vi "Read AJ error Info Table.vi"(8 "error in (no error)":errorcluster, 10 "s":bool, 11 "Linename":string) -> (0 "error IO":errorcluster, 1 "size(s)":i32, 2 "Error BG":u32(colorbox), 3 "Array":string[](array[string]))   [LabVIEW 2014]
uses:
  <vilib>/addons/database/NI_Database_API.lvlib
  <vilib>/addons/database/Connection.llb/DB Tools Open Connec (String).vi
  <vilib>/addons/database/_DB Variant To Data/Database Variant To Data.xnode
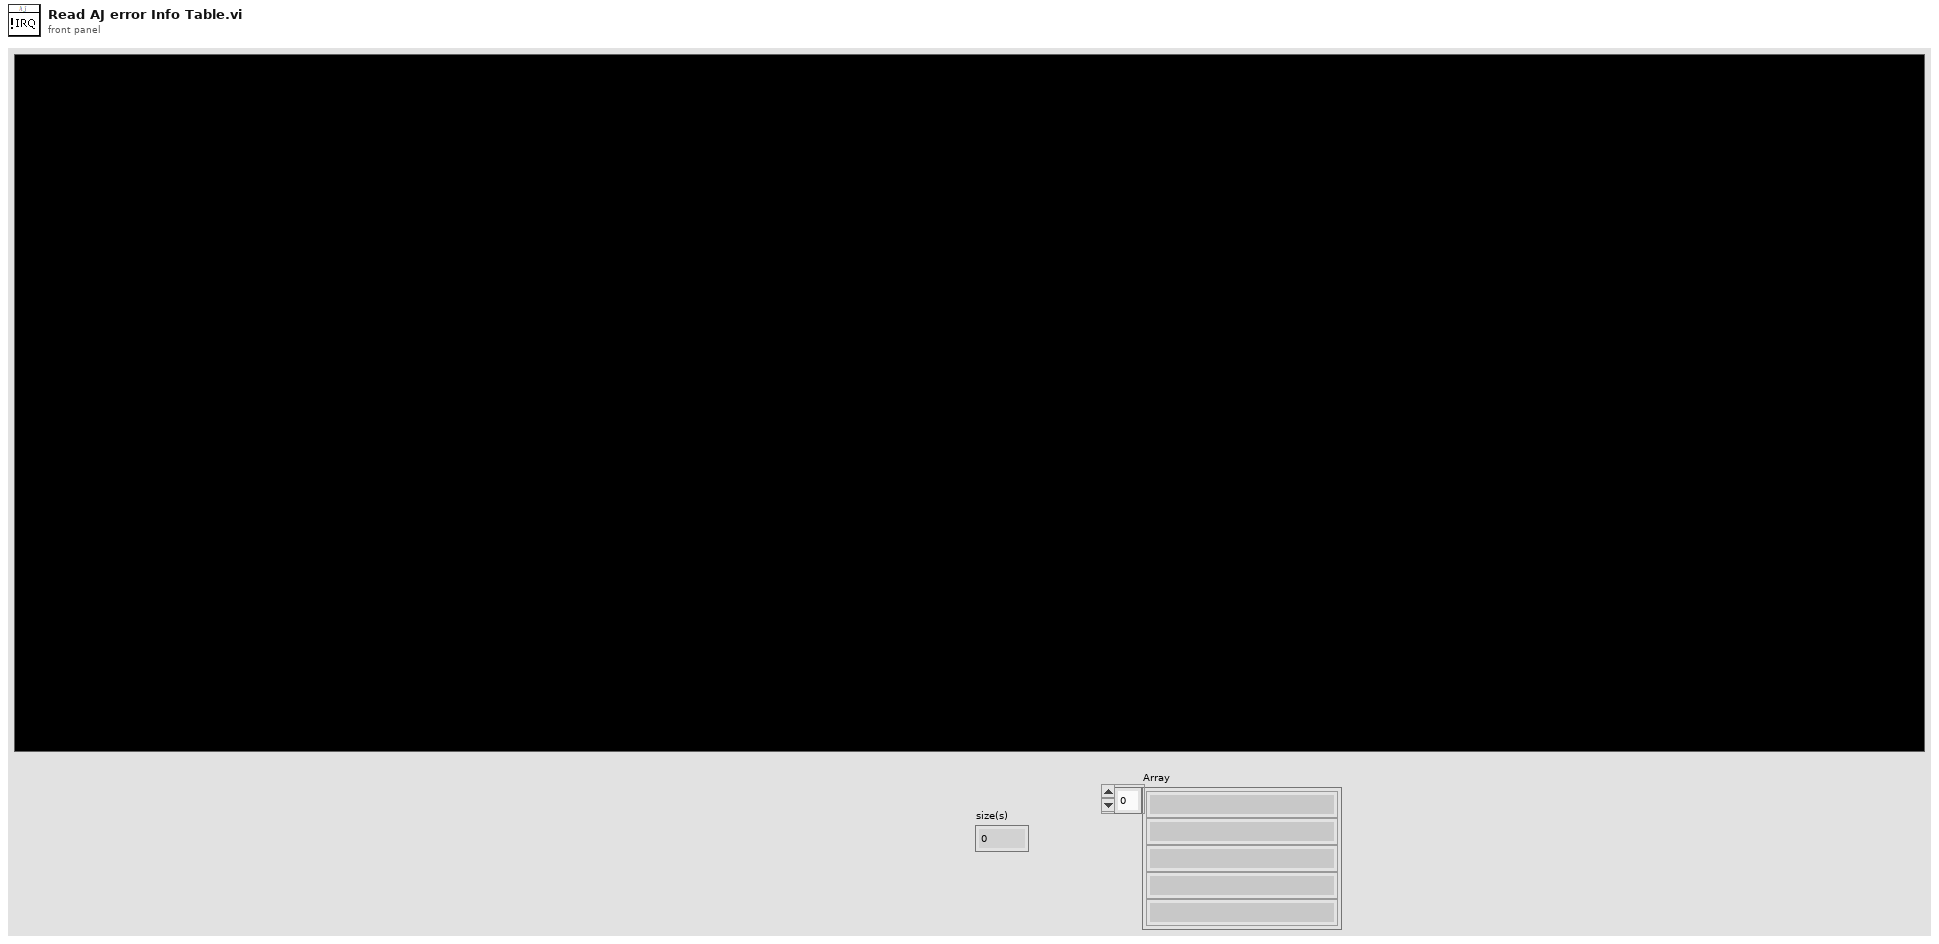
[diagram p1: front panel]
types:
  T1 = cluster{"linename":string, "Stationname":string, "Display Info":string, "startTime":timestamp}[]
  T2 = typedef "NI_Database_API.lvlib/Conn ObjectReference.ctl" = refnum<k1>
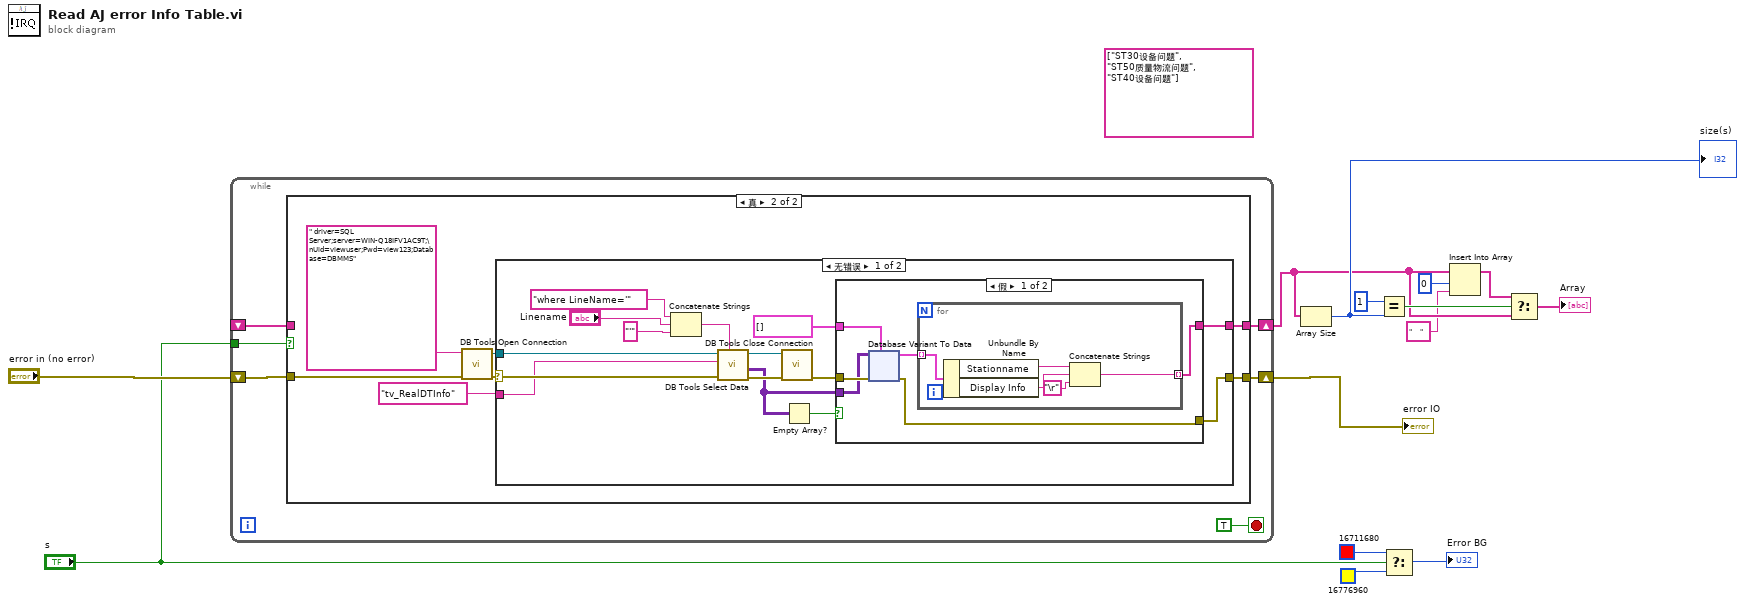
[diagram p0: block diagram]
diagram:
  (unwired) string[] ["ST30设备问题", "ST50质量物流问题", "ST40设备问题"]
  n1 = while {
    tunnel: "s" -> [w15]
    shift-right: [w19] -> w10
    shift-left: "error in (no error)" -> [w20]
    shift-right: [w18] -> w2
    shift-left: _ -> [w16]
    stop <- TRUE stop-if-true
    n2 = case shown="真" w15 {
      tunnel: w20 -> [w21 w28]
      tunnel: [w21 w27] -> w19
      tunnel: [w22 w23] -> w18
      tunnel: w16 -> [w22 _]
      frame False {
      }
      frame True {
        n3 = call-poly <vilib>:"DB Tools Open Connection.vi"("error in (no error)"=w28, "connection information"=" driver=SQL Server;server=WIN-Q18IFV1AC9T;\nUid=viewuser;Pwd=view123;Database=DBMMS") -> ("error out"=w25:errorcluster, "connection reference"=w26:T2)  [unwired: 6 in]
        n4 = case shown="无错误" w25 {
          selector: w25 -> [w43 w204]
          tunnel: w26 -> [w44 _]
          tunnel: "tv_RealDTInfo" ("table") -> [w42 _]
          tunnel: [w31 w204] -> w27
          tunnel: [w30 _] -> w23
          frame No Error {
            n5 = Concatenate Strings("where LineName='", "Linename", "'" ("string")) -> (w37:string)
            n6 = call <vilib>:"DB Tools Select Data.vi"("condition"=w37, "error in (no error)"=w43, "table"=w42, "connection reference"=w44) -> ("error out"=w36:errorcluster, "data"=w33:variant[][], "connection reference out"=w41:T2)  [unwired: 2 in]
            n7 = call <vilib>:"DB Tools Close Connection.vi"("error in (no error)"=w36, "connection reference"=w41) -> ("error out"=w34:errorcluster)  [unwired: 5 in]
            n8 = Empty Array?(array=w33) -> (empty?=w35:bool)
            n9 = case shown="假" w35 {
              tunnel: w34 -> [w50 w203]
              tunnel: w33 -> [w49 _]
              tunnel: T1 [] -> [w48 _]
              tunnel: [w47 w203] -> w31
              tunnel: [w45 _] -> w30
              frame False {
                n10 = xnode "Database Variant To Data"("database variant"=w49, "error in (no error)"=w50, "type"=w48) -> ("data"=w46:T1, "error out"=w47:errorcluster)
                n11 = for {
                  tunnel: w46 -> [w55] mode=indexing
                  tunnel: [w51] -> w45 mode=indexing
                  n12 = Unbundle By Name(w55) -> ("Stationname"=w54:string, "Display Info"=w53:string)
                  n13 = Concatenate Strings(w54, w53, "\r") -> (w51:string)
                }
              }
              frame True {
              }
            }
          }
          frame Error {
          }
        }
      }
    }
  }
  "error IO" <- w10
  n14 = Array Size(array=w2) -> (size(s)=w8:i32)
  "size(s)" <- w8
  n15 = Equal?(x=1, y=w8) -> (x = y?=w6:bool)
  n16 = Select(t=u32 16711680, s="s", f=u32 16776960) -> (s? t:f=→"Error BG":u32)
  n17 = Insert Into Array(array=w2, index=0, new element="    ") -> (w3:string[])
  n18 = Select(t=w3, s=w6, f=w2) -> (s? t:f=→"Array":string[])
